vi "Handle Command.vi"(8 "error in (no error)":errorcluster, 9 "Data":variant, 10 "Command":string, 11 "Example Instrument in":refnum<class "Instrument.Framework-Template.lvclass">) -> (0 "error out":errorcluster, 1 "Processed Data":variant, 2 "Command":string, 3 "Example Instrument out":refnum<class "Instrument.Framework-Template.lvclass">)   [LabVIEW 2019, in "Instrument.Framework-Template.lvclass"]
uses:
  Instrument.Framework-Template.lvclass
  Instrument.Framework-Template.lvclass/Instrument.Framework-Template.ctl
  7d5c8d57-f0a0-4908-8abf-1b878744cce4.vi
  7d5c8d57-f0a0-4908-8abf-1b878744cce4.vi/21baf2a5-a05e-4040-abb6-e44bfa6fb438.vi
  7d5c8d57-f0a0-4908-8abf-1b878744cce4.vi/2a9e1cf6-f0cb-4205-b2a2-302e5ae42f7a.vi
  <vilib>/Utility/Data Type/Get Type Information.vi
  <vilib>/JDP Science/JSONtext/JSON text to Variant.vi
  <vilib>/JDP Science/JSONtext/LVClass Serializer/JSONtext LVClass Serializer.lvclass
  Framework/Instrument Types/SCPI/Instrument.SCPI.lvclass
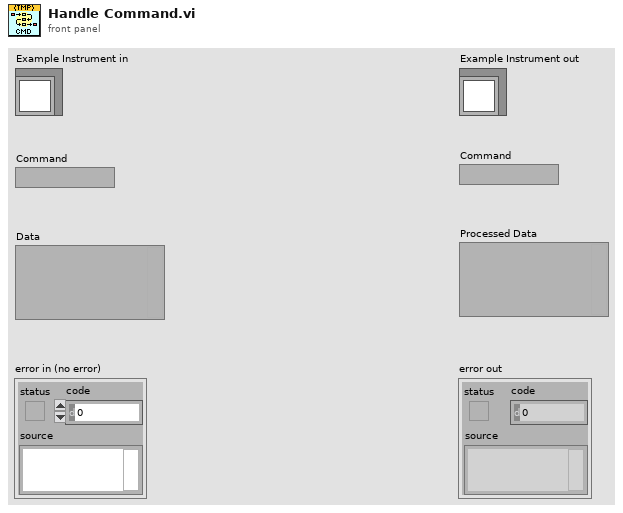
[diagram p1: front panel]
types:
  T1 = typedef "Instrument.Framework-Template.lvclass/Instrument.Framework-Template.getAll--Cluster.ctl" = cluster{"Levy 1":dbl, "Logger SMO":dbl, "SMO Boolean":bool, "SMO String":string}
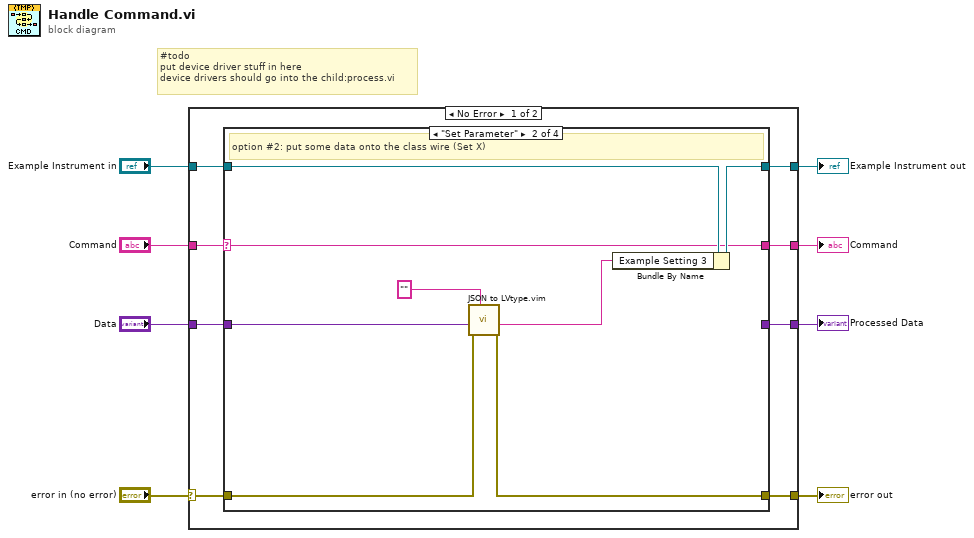
[diagram p0: block diagram]
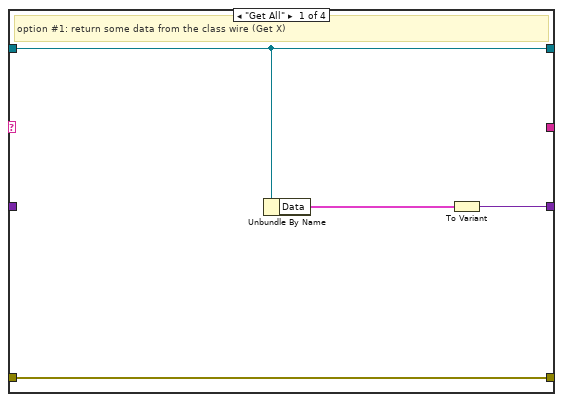
[diagram p2: hidden frame]
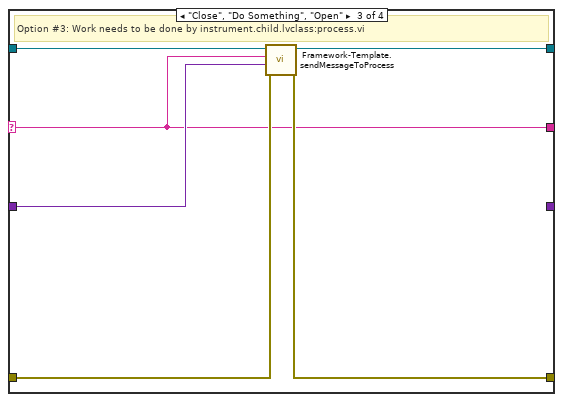
[diagram p3: hidden frame]
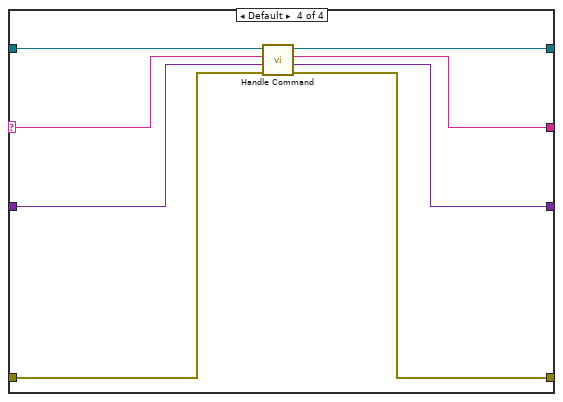
[diagram p4: hidden frame]
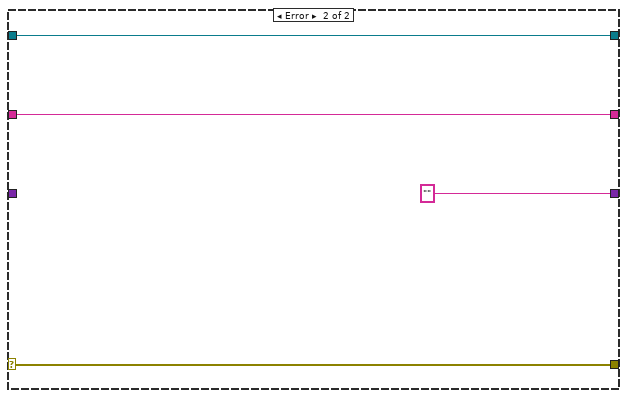
[diagram p5: hidden frame]
diagram:
  # "#todo\nput device driver stuff in here\ndevice drivers should go into the child:process.vi"
  n1 = case shown="No Error" "error in (no error)" {
    selector: "error in (no error)" -> [w10 w46]
    tunnel: [w12 w46] -> w6
    tunnel: [w14 w45] -> w5
    tunnel: "Example Instrument in" -> [w15 w45]
    tunnel: "Command" -> [w16 w43]
    tunnel: [w13 "" ("String")] -> w3
    tunnel: "Data" -> [w9 _]
    tunnel: [w11 w43] -> w1
    frame No Error {
      n2 = case shown="\"Set Parameter\"" w16 {
        selector: w16 -> [_ w23 w29 w36]
        tunnel: w15 -> [w19 w28 w34 w40]
        tunnel: [w19 w27 w33 w37] -> w14
        tunnel: [w17 _ _ w39] -> w13
        tunnel: w10 -> [w18 w26 w32 w41]
        tunnel: w9 -> [_ w24 w30 w42]
        tunnel: [w18 w25 w31 w38] -> w12
        tunnel: [_ w23 w29 w35] -> w11
        frame "Get All" {
          # "option #1: return some data from the class wire (Get X)"
          n3 = Unbundle By Name(w19) -> ("Data"=w20:T1)
          n4 = To Variant(anything=w20) -> (Variant=w17:variant)
        }
        frame "Set Parameter" {
          # "option #2: put some data onto the class wire (Set X)"
          n5 = call "JSON to LVtype.vim"("type"="", "error in (no error)"=w26, "JSON Data in"=w24) -> ("error out"=w25:errorcluster, "Data out"=w22:string)  [unwired: 7 in]
          n6 = Bundle By Name(cluster=w28, "Example Setting 3"=w22) -> (w27:refnum<class "Instrument.Framework-Template.lvclass">)
        }
        frame "Close", "Do Something", "Open" {
          # "Option #3: Work needs to be done by instrument.child.lvclass:process.vi"
          n7 = call "Framework-Template.sendMessageToProcess.vi"("error in (no error)"=w32, "Data"=w30, "Command"=w29, "Framework-Template in"=w34) -> ("error out"=w31:errorcluster, "Framework-Template out"=w33:refnum<class "Instrument.Framework-Template.lvclass">)  [unwired: 6 in]
        }
        frame Default {
          n8 = call-parent "Handle Command.vi"("error in (no error)"=w41, "Data"=w42, "Command"=w36, "Instrument in"=w40) -> ("error out"=w38:errorcluster, "Processed Data"=w39:variant, "Command"=w35:string, "Instrument out"=w37:refnum<class "Instrument.Framework-Template.lvclass">)  [unwired: 4 in]
        }
      }
    }
    frame Error {
    }
  }
  "error out" <- w6
  "Example Instrument out" <- w5
  "Command" <- w1
  "Processed Data" <- w3
